vi "vi locker.vi"() -> ()   [LabVIEW 2013]
panel:
  out "error out":errorcluster
  in  "Path":path=path "C:/"
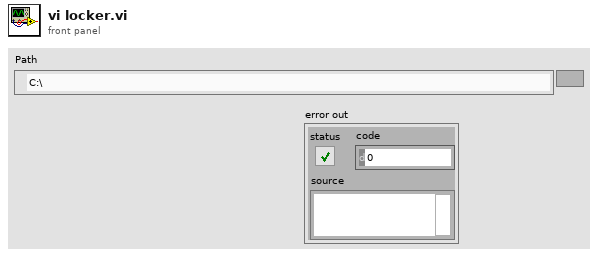
[diagram p1: front panel]
types:
  T1 = enum32{"invalid lock state", "Not Locked", "Locked (No Password)", "Password-protected"}
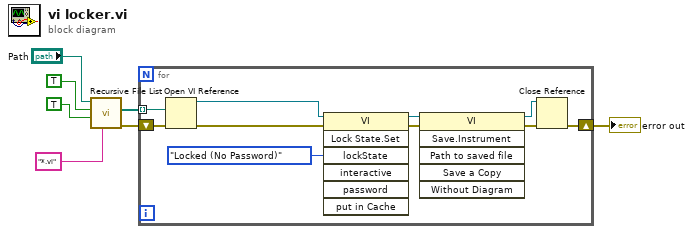
[diagram p0: block diagram]
diagram:
  n1 = call <vilib>:"Recursive File List.vi"("pattern"="*.vi", "Continue Recursing on Error? (F)"=TRUE, "Treat LLBs as Folders?"=TRUE, "Folder Path"="Path") -> ("error out"=w3:errorcluster, "All Files in Dir"=w2:path[])  [unwired: 3 in, 3 out]
  n2 = for {
    shift-right: [w15] -> w1
    shift-left: w3 -> [w17]
    tunnel: w2 -> [w16] mode=indexing
    n3 = Open VI Reference(vi path=w16, error in (no error)=w17) -> (vi reference=w12:refnum<vi>, error out=w11:errorcluster)  [unwired: 4 in]
    n4 = invoke class="VI" method="Lock State.Set"(reference=w12, error in=w11, "lockState"=T1."Locked (No Password)" ("Lock State")) -> (reference out=w10:refnum<vi>, error out=w9:errorcluster)  [unwired: 4 in, 5 out]
    n5 = invoke class="VI" method="Save.Instrument"(reference=w10, error in=w9) -> (reference out=w13:refnum<vi>, error out=w14:errorcluster)  [unwired: 4 in, 4 out]
    n6 = Close Reference(reference=w13, error in (no error)=w14) -> (error out=w15:errorcluster)
  }
  "error out" <- w1
